vi "Sensor Ref Curve Leveling.vi"(8 "error in (no error)":errorcluster caption="错误输入（无错误）", 9 "refOffset":dbl, 10 "autoOffsetCorrection":i32, 11 "sensorHandle":i32) -> (0 "error out":errorcluster caption="错误输出", 3 "function return":i32)   [LabVIEW 2018]
doc: "extern int __stdcall APSxSensorRefCurveLeveling (int sensorHandle, IN int autoOffsetCorrection, IN double refOffset);"
uses:
  APSx.dll/APSx.dll
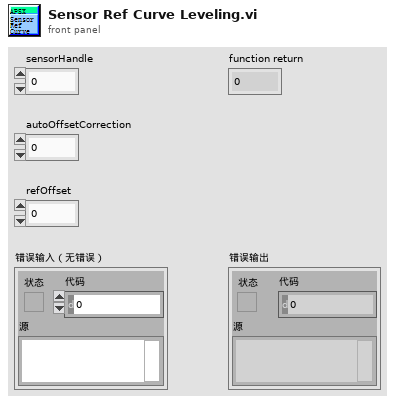
[diagram p1: front panel]
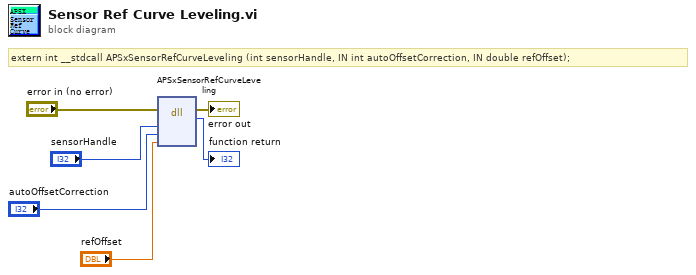
[diagram p0: block diagram]
diagram:
  # "extern int __stdcall APSxSensorRefCurveLeveling (int sensorHandle, IN int autoOffsetCorrection, IN double refOffset);"
  n1 = dll-call lib="PTH2[abs D项目Feng恒隆项目Labview传感器对中台SourcesAPSx.dllAPSx.*" fn="APSxSensorRefCurveLeveling"(error in="error in (no error)", "sensorHandle"="sensorHandle", "autoOffsetCorrection"="autoOffsetCorrection", "refOffset"="refOffset") -> (error out=→"error out":errorcluster, →"function return":i32)  [unwired: 5 in, 1 out]
